vi "NewPower_FormatCurrentt.vi"(2 "y":dbl, 3 "FetchStr":string) -> (0 "Current":dbl)   [LabVIEW 2015]
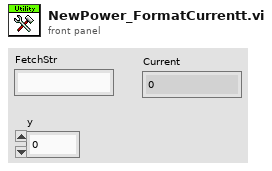
[diagram p1: front panel]
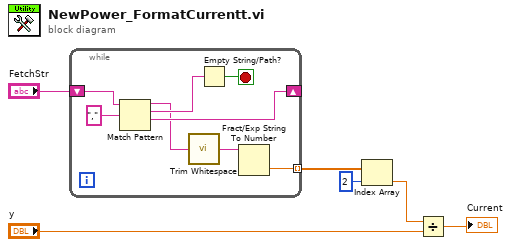
[diagram p0: block diagram]
diagram:
  n1 = while {
    shift-right: [w10] -> _
    shift-left: "FetchStr" -> [w14]
    tunnel: [w7] -> w5 mode=indexing
    stop <- w12 stop-if-true
    n2 = Match Pattern(string=w14, regular expression=",") -> (before substring=w9:string, match substring=w11:string, after substring=w10:string)  [unwired: 1 in, 1 out]
    n3 = call <vilib>:"Trim Whitespace.vi"("string"=w9) -> ("trimmed string"=w8:string)  [unwired: 1 in]
    n4 = Empty String/Path?(string/path=w11) -> (empty?=w12:bool)
    n5 = Fract/Exp String To Number(string=w8) -> (number=w7:dbl)  [unwired: 3 in, 1 out]
  }
  n6 = Index Array(array=w5, index=2) -> (element=w3:dbl)
  n7 = Divide(x=w3, y="y") -> (x/y=→"Current":dbl)
